vi "List Available Cameras.vi"(8 "error in":errorcluster) -> (0 "error out":errorcluster, 2 "VendorName":string[](array[string]), 3 "Available Cameras":string[](array[string]))   [LabVIEW 2024]
doc: "Lista wszystkich kamer, które zostały skonfigurowane w MAX"
uses:
  <vilib>/vision/driver/NI_Vision_Acquisition_Software.lvlib
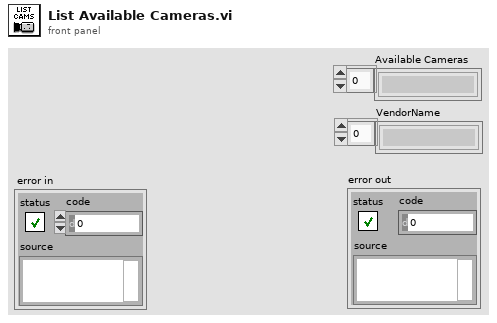
[diagram p1: front panel]
types:
  T1 = cluster{"Type":u32, "Version":u32, "Flags":u32, "SerialNumberHigh":u32, "SerialNumberLow":u32, "BusType":u32, "InterfaceName":string, "VendorName":string, "ModelName":string, "CameraFileName":string, "CameraAttributeURL":string}[]
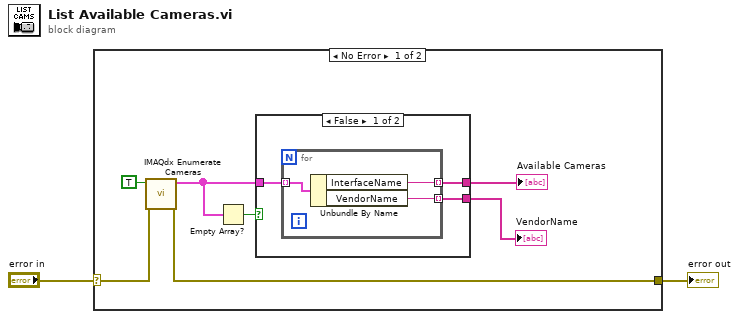
[diagram p0: block diagram]
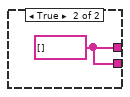
[diagram p2: hidden frame]
diagram:
  n1 = case shown="No Error" "error in" {
    selector: "error in" -> [w4 w17]
    tunnel: [w3 w17] -> w1
    frame No Error {
      n2 = call <vilib>:"IMAQdx Enumerate Cameras.vi"("error in"=w4, "Connected Only? (Yes)"=TRUE) -> ("error out"=w3:errorcluster, "Camera Information Array"=w7:T1)  [unwired: 8 in]
      n3 = Empty Array?(array=w7) -> (empty?=w8:bool)
      n4 = case shown="False" w8 {
        tunnel: w7 -> [w12 _]
        tunnel: [w11 w16] -> w5
        tunnel: [w10 w16] -> w6
        frame False {
          n5 = for {
            tunnel: w12 -> [w15] mode=indexing
            tunnel: [w14] -> w11 mode=indexing
            tunnel: [w13] -> w10 mode=indexing
            n6 = Unbundle By Name(w15) -> ("InterfaceName"=w14:string, "VendorName"=w13:string)
          }
        }
        frame True {
          w16 = string[] []
        }
      }
      "VendorName" <- w6
      "Available Cameras" <- w5
    }
    frame Error {
    }
  }
  "error out" <- w1
